vi "Header_PS.vi"(8 "error in":errorcluster, 11 "Headers In":cluster{"Name":string, "Value":string}[](array[cluster])) -> (0 "error out":errorcluster, 3 "Headers_PS_Dict":string)   [LabVIEW 2020, in "Request.lvclass"]
uses:
  Request.lvclass
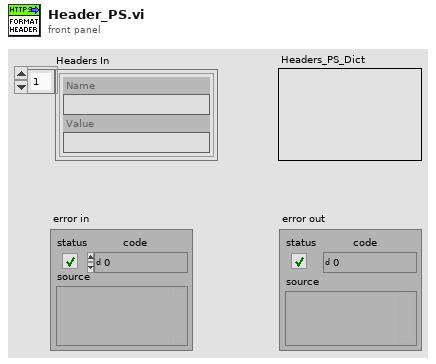
[diagram p1: front panel]
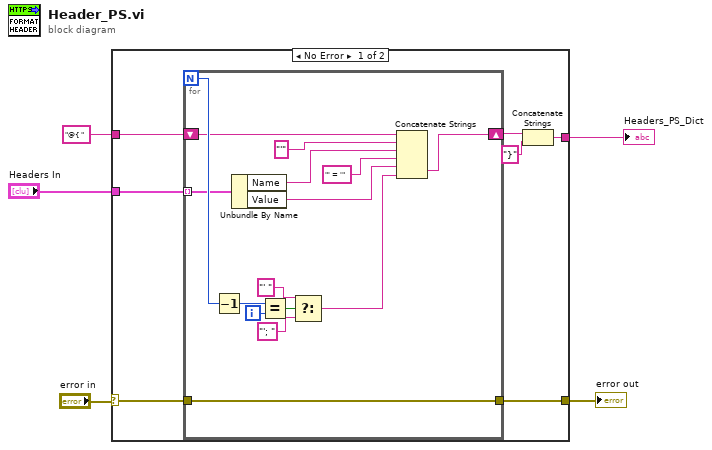
[diagram p0: block diagram]
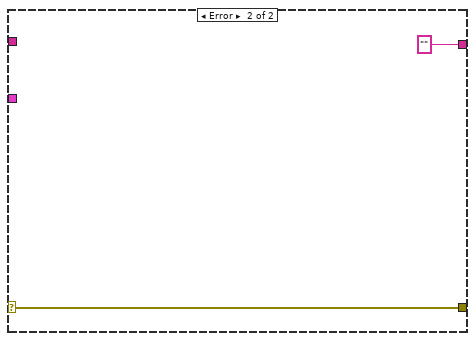
[diagram p2: hidden frame]
diagram:
  n1 = case shown="No Error" "error in" {
    selector: "error in" -> [w12 w28]
    tunnel: [w11 w28] -> w4
    tunnel: "Headers In" -> [w10 _]
    tunnel: "@{ " -> [w9 _]
    tunnel: [w6 ""] -> w1
    frame No Error {
      n2 = for {
        N -> [w25]
        tunnel: w12 -> [w27]
        tunnel: [w27] -> w11
        tunnel: w10 -> [w20] mode=indexing
        shift-right: [w14] -> w8
        shift-left: w9 -> [w13]
        i -> [w24]
        n3 = Decrement(x=w25) -> (x-1=w23:i32)
        n4 = Unbundle By Name(w20) -> ("Name"=w18:string, "Value"=w16:string)
        n5 = Equal?(x=w23, y=w24) -> (x = y?=w26:bool)
        n6 = Select(t="' ", s=w26, f="'; ") -> (s? t:f=w15:string)
        n7 = Concatenate Strings(w13, "'" ("string"), w18, "' = '" ("string"), w16, w15) -> (w14:string)
      }
      n8 = Concatenate Strings(w8, "}" ("string")) -> (w6:string)
    }
    frame Error {
    }
  }
  "error out" <- w4
  "Headers_PS_Dict" <- w1
